vi "Average_Buffer.vi"(3 "N_Elements":i32, 4 "Index":u64, 5 "Buffersize":i32, 6 "Buffer in":T2(array[cluster])) -> (1 "output devs":T1, 2 "output means":T1)   [LabVIEW 2009]
uses:
  <vilib>/Analysis/NI_AALBase.lvlib
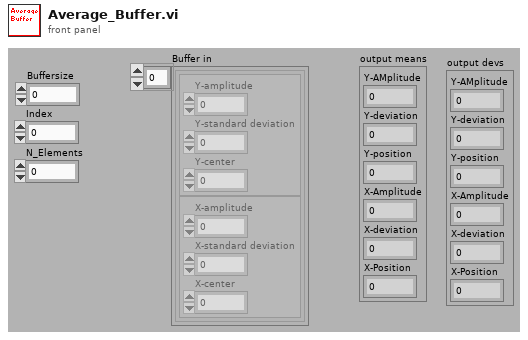
[diagram p1: front panel]
types:
  T1 = cluster{"Y-AMplitude":dbl, "Y-deviation":dbl, "Y-position":dbl, "X-Amplitude":dbl, "X-deviation":dbl, "X-Position":dbl}
  T2 = cluster{cluster{"Y-amplitude":dbl, "Y-standard deviation":dbl, "Y-center":dbl}, cluster{"X-amplitude":dbl, "X-standard deviation":dbl, "X-center":dbl}}[]
  T3 = cluster{cluster{"Y-amplitude":dbl, "Y-standard deviation":dbl, "Y-center":dbl}, cluster{"X-amplitude":dbl, "X-standard deviation":dbl, "X-center":dbl}}
  T4 = cluster{"Y-amplitude":dbl, "Y-standard deviation":dbl, "Y-center":dbl}
  T5 = cluster{"X-amplitude":dbl, "X-standard deviation":dbl, "X-center":dbl}
  T6 = cluster{"mean":dbl, "mean":dbl, "mean":dbl, "mean":dbl, "mean":dbl, "mean":dbl}
  T7 = cluster{"standard deviation":dbl, "standard deviation":dbl, "standard deviation":dbl, "standard deviation":dbl, "standard deviation":dbl, "standard deviation":dbl}
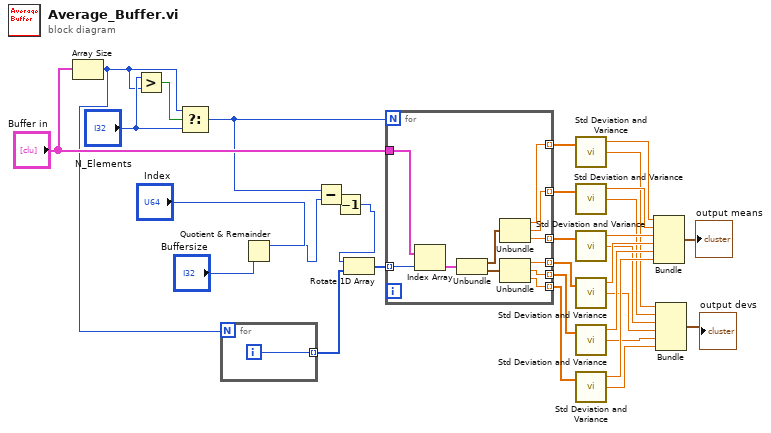
[diagram p0: block diagram]
diagram:
  n1 = Array Size(array="Buffer in") -> (size(s)=w5:i32)
  n2 = Greater?(x="N_Elements", y=w5) -> (0:w19:bool)
  n3 = Select(t=w5, s=w19, f="N_Elements") -> (s? t:f=w4:i32)
  n4 = for {
    N: w5 -> [_]
    tunnel: [w33] -> w15 mode=indexing
    i -> [w33]
  }
  n5 = Quotient & Remainder(x="Index", y="Buffersize") -> (x-y*floor(x/y)=w3:u64)  [unwired: 1 out]
  n6 = Subtract(x=w4, y=w3) -> (x-y=w2:u64)
  n7 = Decrement(x=w2) -> (x-1=w1:u64)
  n8 = Rotate 1D Array(1:w15, 2:w1) -> (0:w13:i32[])
  n9 = for {
    N: w4 -> [_]
    tunnel: [w42] -> w31 mode=indexing
    tunnel: [w41] -> w30 mode=indexing
    tunnel: [w40] -> w29 mode=indexing
    tunnel: [w39] -> w28 mode=indexing
    tunnel: [w38] -> w27 mode=indexing
    tunnel: [w37] -> w26 mode=indexing
    tunnel: "Buffer in" -> [w36]
    tunnel: w13 -> [w34] mode=indexing
    n10 = Index Array(array=w36, index=w34) -> (element=w35:T3)
    n11 = Unbundle(w35) -> (w44:T4, w43:T5)
    n12 = Unbundle(w44) -> ("Y-amplitude"=w42:dbl, "Y-standard deviation"=w41:dbl, "Y-center"=w40:dbl)
    n13 = Unbundle(w43) -> ("X-amplitude"=w39:dbl, "X-standard deviation"=w38:dbl, "X-center"=w37:dbl)
  }
  n14 = call <vilib>:"Std Deviation and Variance.vi"("X"=w31) -> ("mean"=w25:dbl, "standard deviation"=w12:dbl)  [unwired: 1 in, 1 out]
  n15 = call <vilib>:"Std Deviation and Variance.vi"("X"=w30) -> ("mean"=w24:dbl, "standard deviation"=w11:dbl)  [unwired: 1 in, 1 out]
  n16 = call <vilib>:"Std Deviation and Variance.vi"("X"=w29) -> ("mean"=w23:dbl, "standard deviation"=w10:dbl)  [unwired: 1 in, 1 out]
  n17 = call <vilib>:"Std Deviation and Variance.vi"("X"=w28) -> ("mean"=w22:dbl, "standard deviation"=w9:dbl)  [unwired: 1 in, 1 out]
  n18 = call <vilib>:"Std Deviation and Variance.vi"("X"=w27) -> ("mean"=w21:dbl, "standard deviation"=w8:dbl)  [unwired: 1 in, 1 out]
  n19 = call <vilib>:"Std Deviation and Variance.vi"("X"=w26) -> ("mean"=w20:dbl, "standard deviation"=w7:dbl)  [unwired: 1 in, 1 out]
  n20 = Bundle("mean"=w25, "mean"=w24, "mean"=w23, "mean"=w22, "mean"=w21, "mean"=w20) -> (→"output means":T6)  [unwired: 1 in]
  n21 = Bundle("standard deviation"=w12, "standard deviation"=w11, "standard deviation"=w10, "standard deviation"=w9, "standard deviation"=w8, "standard deviation"=w7) -> (→"output devs":T7)  [unwired: 1 in]
